vi "mod_Resample (complex).vi"(0 "x":cdb[](array[numeric]) format="%.2f", 5 "config":T1={"new sample period"=0.0, "Timing Jitter"=enum."Interpolation", "first point location"=0.0, "prototype filter"={"h"=[], "Max Decimation"=1024.0}} {"prototype filter"."h" format="%.2f"; "prototype filter"."Max Decimation" format="%.2f"; "first point location" format="%.2f"; "new sample period" format="%.2f"}, 13 "Reset? (T)":bool=TRUE, 14 "flush buffers? (F)":bool) -> (4 "y":cdb[](array[numeric]) format="%.2f", 15 "error out":errorcluster)   [LabVIEW 2020, in "niAMT.lvlib"]
uses:
  <vilib>/addons/Modulation/niAMT.lvlib
  <vilib>/addons/Modulation/Analog/support/mod_PerformResampling.vi
  <vilib>/addons/Modulation/Analog/support/mod_ResamplingFilter.vi
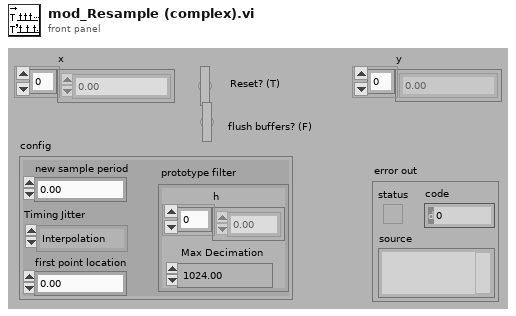
[diagram p1: front panel]
types:
  T1 = cluster{"new sample period":dbl, "Timing Jitter":enum32{"Interpolation", "Rounding"}, "first point location":dbl, "prototype filter":cluster{"h":dbl[], "Max Decimation":dbl}}
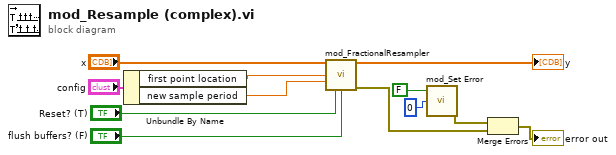
[diagram p0: block diagram]
diagram:
  n1 = Unbundle By Name("config") -> ("first point location"=w7:dbl, "new sample period"=w1:dbl)
  n2 = call <vilib>:"mod_FractionalResampler.vi"("samples in"="x", "offset"=w7, "rate factor"=w1, "reset"="Reset? (T)", "flush"="flush buffers? (F)") -> ("samples out"=→"y":cdb[], "error out"=w3:errorcluster)  [unwired: 1 in, 8 out]
  n3 = call <vilib>:"mod_Set Error.vi"("code"=0, "status"=FALSE) -> ("error out"=w4:errorcluster)  [unwired: 6 out]
  n4 = Merge Errors(w4, w3) -> (→"error out":errorcluster)
